vi "AprilTag RoboRIO.vi"() -> ()   [LabVIEW 2023]
uses:
  filter Selector.ctl
  <vilib>/Rock Robotics/WPI/Camera/WPI_CameraImageSize.ctl
  <vilib>/Analysis/baseanly.llb/Real Inverse Matrix.vi
  <vilib>/Analysis/NI_AALBase.lvlib
panel:
  in  "Hilite":bool=TRUE
  in  "Draw Visuals":bool=TRUE
  out "Instructions:":string="Run the VI using the run arrow above. Choose a camera or provided file. Update the tag family to search for. You can change camera resolution on the diagram, outside the loop.\n\nExplore and follow the AprilTag tutorial to explore accuracy and performance tradeoffs. Real-world distance and orientation measurements require tuning the scaling and intrinsic camera matrix beneath the image.\n\nThe white picture to the right is a birds-eye view of a robot with a front-facing camera. The 3D origin is shown at the top-center of the field where the apriltag is attached to that wall.  The charts farther to the right show the YPR and XYZ derived measurements in degrees and inches. Still farther is the detailed info (ID, pixel info, score, and homography matrix)."
  in  "Hamming cutoff":i32
  in  "filter":T1
  out "Y (in)":dbl format="%.1f"
  out "Z (in)":dbl format="%.1f"
  out "X (in)":dbl format="%.1f"
  in  "Length (in)":dbl=100.0
  in  "width (in)":dbl=100.0
  out "Picture":picture
  in  "show rejects":bool
  out "bad":i32
  out "loop time (s)":dbl
  in  "Scale to Inches":dbl[](array[numeric])=[2.5, 2.5, 2.5]
  out "YPR (deg)":cluster{"yaw":dbl, "pitch":dbl, "roll":dbl} {"yaw" format="%.1f"; "pitch" format="%.1f"; "roll" format="%.1f"}
  out "ofsets (in)":cluster{"X":dbl, "Y":dbl, "Z":dbl} {"X" format="%.1f"; "Y" format="%.1f"; "Z" format="%.1f"}
  in  "Intrinsic Camera Matrix":dbl[][](array[numeric])=[[1135.0, 0.0, 640.0], [0.0, 1135.0, 360.0], [0.0, 0.0, 1.0]]
  out "good":i32
  in  "Tag Familys":string[](array[combo])=["16h5"]
  in  "blur":dbl step=0.1
  in  "refine Edges":bool=TRUE
  in  "decimate":dbl=4.0
  in  "threads":i32=1
  out "search time (s)":dbl
  out "good tag details":T2(array[cluster])
  in  "score cutoff":dbl(slide)=60.60606060606061 scale=0.0..100.0
  out "Image":T3(plugin-control)
  # "Offset between\ntarget and camera"
  # "Angles between\ntarget and camera"
  # "Better way to pick camera matrix\ncheck other cams and simplify scaling"
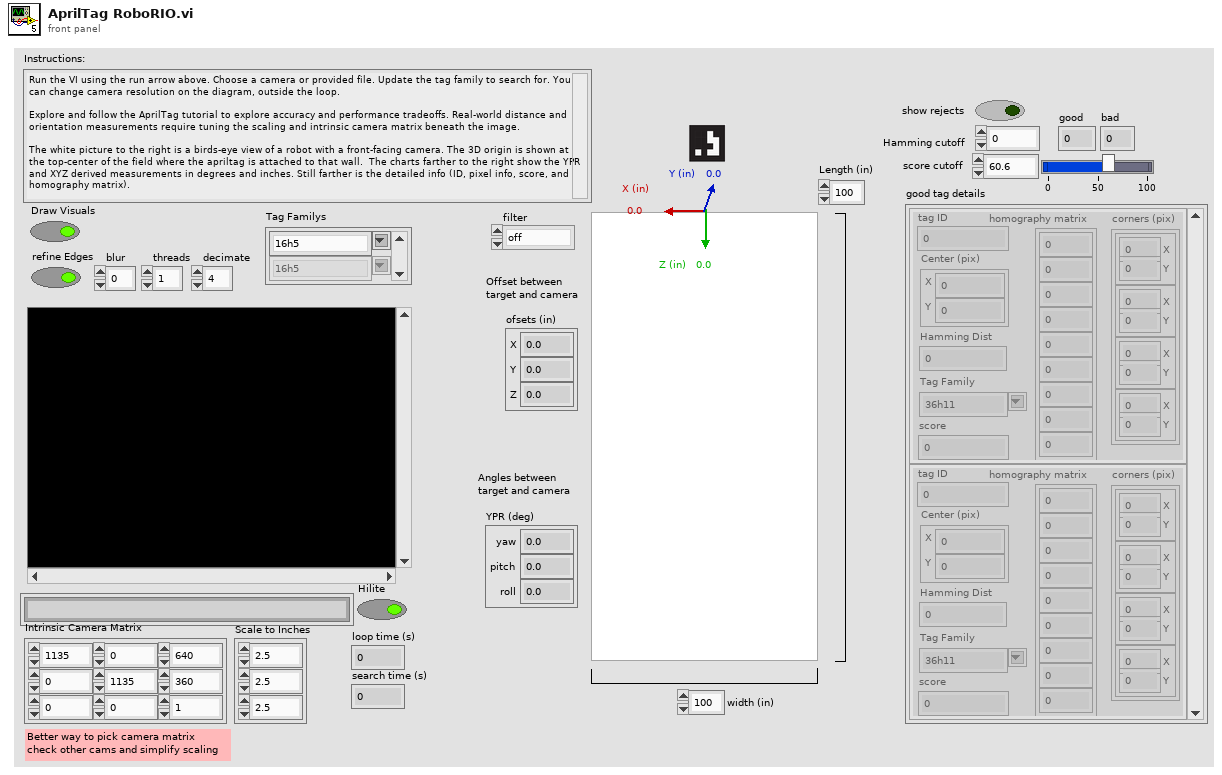
[diagram p1: front panel]
types:
  T1 = typedef "filter Selector.ctl" = enum16{"off", "2 pt avg", "low pass"}
  T2 = cluster{"tag ID":i32, "Center (pix)":cluster{"X":dbl, "Y":dbl}, "homography matrix":dbl[], "score":dbl, "Hamming Dist":i32, "corners (pix)":cluster{"X":dbl, "Y":dbl}[], "Tag Family":string}[]
  T3 = typedef "IMAQ Image.ctl" = refnum<image>
  T4 = typedef "WPI_CameraImageSize.ctl" = enum16{"640x480", "320x240", "160x120", "Custom"}
  T5 = typedef "Image Type" = u32
  T6 = typedef "WPI_CameraDevRef.ctl" = cluster{"Camera Address":string, "CameraStatus":errorcluster}
  T7 = cluster{"tag ID":i32, "Center":cluster{"X":dbl, "Y":dbl}, "homography matrix":dbl[], "decision margin":dbl, "Hamming Dist":i32, "corner points":cluster{"X":dbl, "Y":dbl}[], "Tag Family":string}[]
  T8 = cluster{"Hamming cutoff":i32, "score cutoff":dbl, "show rejects":bool}
  T9 = cluster{"tag ID":i32, "Center":cluster{"X":dbl, "Y":dbl}, "Homography Matrix":dbl[], "dec margin":dbl, "Hamming Dist":i32, "Corner Points":cluster{"X":dbl, "Y":dbl}[], "Tag Family":string}[]
  T10 = typedef "NI_Matrix.lvlib/RealMatrix.ctl" = dbl[][]
  T11 = typedef "LVBoundsTypeDef.ctl" = cluster{"Width":u32, "Height":u32}
  T12 = cluster{"tag ID":i32, "Center":cluster{"X":dbl, "Y":dbl}, "Homography Matrix":dbl[], "dec margin":dbl, "Hamming Dist":i32, "Corner Points":cluster{"X":dbl, "Y":dbl}[], "Tag Family":string}
  T13 = cluster{"Translation[0]":dbl, "Translation[1]":dbl, "Translation[2]":dbl}
  T14 = cluster{"picture out":picture, "offset":cluster{dbl, dbl}}
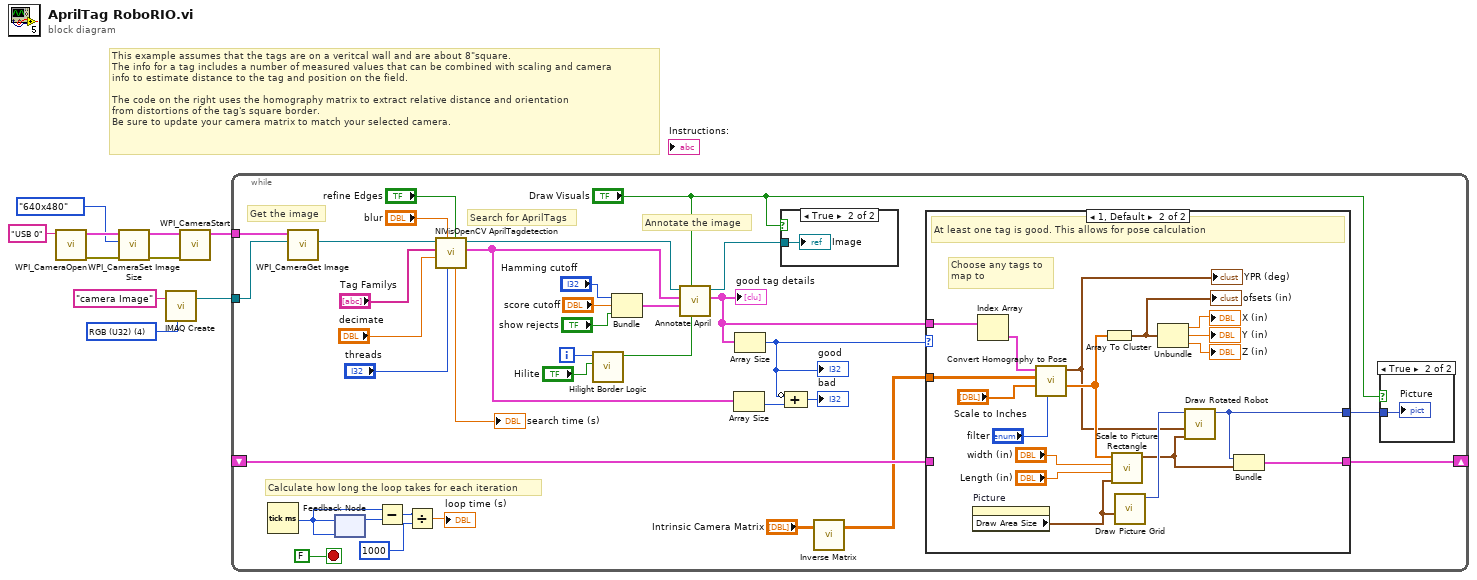
[diagram p0: block diagram]
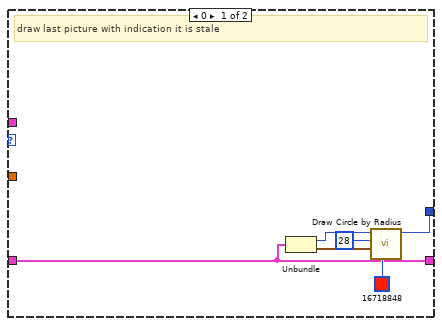
[diagram p4: hidden frame]
diagram:
  w7 = T5 4 items=["Grayscale (U8)", "Grayscale (I16)", "Grayscale (SGL)", "Complex (CSG)", "RGB (U32)", "HSL (U32)", "RGB (U64)", "Grayscale (U16)"] ("Image Type")
  # "This example assumes that the tags are on a veritcal wall and are about 8\"square. \nThe info for a tag includes a number of measured values that can be combined with scaling and camera\ninfo to estimate distance to the tag and position on the field. \n\nThe code on the right uses the homography matrix to extract relative distance and orientation\nfrom distortions of the tag's square border.\nBe sure to update your camera matrix to match your selected camera."
  n1 = call <vilib>:"WPI_CameraOpen.vi"("Camera Address"="USB 0") -> ("error out"=w3:errorcluster, "CameraDevRef"=w5:T6)  [unwired: 9 in]
  n2 = call <vilib>:"WPI_CameraSet Image Size.vi"("error in (no error)"=w3, "Image Size"=WPI_CameraImageSize."640x480", "CameraDevRef"=w5) -> ("error out"=w2:errorcluster, "CameraDevRef Out"=w4:T6)  [unwired: 7 in]
  n3 = call "IMAQ Create"("Image Name"="camera Image", "Image Type"=w7) -> ("New Image"=w6:T3)  [unwired: 3 in, 1 out]
  n4 = call <vilib>:"WPI_CameraStart.vi"("error in (no error)"=w2, "CameraDevRef"=w4) -> ("CameraDevRef"=w9:T6)  [unwired: 8 in, 1 out]
  n5 = while {
    shift-right: [w39] -> _
    shift-left: _ -> [w40]
    tunnel: w9 -> [w15]
    tunnel: w6 -> [w14]
    i -> [w26]
    stop <- FALSE stop-if-true
    # "Calculate how long the loop takes for each iteration"
    # "Annotate the image"
    # "Search for AprilTags"
    # "Get the image"
    n6 = Tick Count (ms)() -> (millisecond timer value=w37:u32)
    n7 = call <vilib>:"WPI_CameraGet Image.vi"("Image"=w14, "CameraDevRef"=w15) -> ("Image Out"=w13:T3)  [unwired: 7 in, 2 out]
    n8 = feedback-in #1(w37) -> ()
    n9 = feedback #1(w37) -> (w38:u32)
    n10 = Subtract(x=w37, y=w38) -> (x-y=w29:u32)
    n11 = Divide(x=w29, y=1000) -> (x/y=→"loop time (s)":dbl)
    n12 = call <vilib>:"NIVisOpenCV AprilTagdetection.vi"("refine Edges"="refine Edges", "threads"="threads", "blur"="blur", "decimate"="decimate", "Tag Familys"="Tag Familys", "Image Src"=w13) -> ("Detected Tags"=w20:T7, "Image Dst Out"=w45:T3, "exec time (s)"=→"search time (s)":dbl)  [unwired: 2 in, 1 out]
    n13 = call "Hilight Border Logic.vi"("Hilight"="Hilite", "index"=w26) -> ("Hilight"=w25:bool)  [unwired: 9 in]
    n14 = Bundle("Hamming cutoff"="Hamming cutoff", "score cutoff"="score cutoff", "show rejects"="show rejects") -> (w21:T8)  [unwired: 1 in]
    n15 = call "Annotate April.vi"("hilight"=w25, "Annotate"="Draw Visuals", "cutoffs"=w21, "Detected Tags"=w20, "Refnum in"=w45) -> ("tags"=w19:T9, "Refnum out"=w44:T3)  [unwired: 4 in, 1 out]
    "good tag details" <- w19
    n16 = Array Size(array=w20) -> (size(s)=w36:i32)
    n17 = Array Size(array=w19) -> (size(s)=w18:i32)
    "good" <- w18
    n18 = case shown="True" "Draw Visuals" {
      tunnel: w44 -> [_ w47]
      frame False {
      }
      frame True {
        "Image" <- w47
      }
    }
    n19 = Compound Arithmetic op=ADD(invert w18, w36) -> (→"bad":i32)
    n20 = call-poly <vilib>:"Inverse Matrix.vi"("Input Matrix"="Intrinsic Camera Matrix") -> ("Inverse Matrix"=w16:T10)  [unwired: 1 in, 1 out]
    n21 = case shown="1, Default" w18 {
      tunnel: w16 -> [_ w71]
      tunnel: [w53 w68] -> w41
      tunnel: w40 -> [w48 _]
      tunnel: [w48 w67] -> w39
      tunnel: w19 -> [_ w66]
      frame 0 {
        # "draw last picture with indication it is stale"
        n22 = Unbundle(w48) -> ("picture out"=w52:picture, "offset"=w51:cluster{dbl, dbl})
        n23 = call <vilib>:"Draw Circle by Radius.vi"("color(black)"=u32 16718848, "pixel center"=w51, "radius"=i16 28, "picture"=w52) -> ("new picture"=w53:picture)  [unwired: 7 in]
      }
      frame 1, Default {
        # "Choose any tags to\nmap to"
        # "At least one tag is good. This allows for pose calculation"
        n24 = property on="Picture" class="Pict"() -> ("Draw Area Size"=w57:T11)  [unwired: 2 in, 2 out]
        n25 = Index Array(array=w66) -> (element=w56:T12)  [unwired: 1 in]
        n26 = call "Convert Homography to Pose.vi"("filter"="filter", "Scale to Inches"="Scale to Inches", "Inverse Camera Matrix"=w71, "tag info"=w56) -> ("Translation"=w58:dbl[], "angles (deg)"=w55:cluster{"yaw":dbl, "pitch":dbl, "roll":dbl})  [unwired: 5 in, 1 out]
        "YPR (deg)" <- w55
        n27 = Array To Cluster(array=w58) -> (cluster=w59:T13)
        "ofsets (in)" <- w59
        n28 = call "Scale to Picture Rectangle.vi"("Draw Area Size"=w57, "Length (in)"="Length (in)", "width (in)"="width (in)", "Translation XYZ"=w58) -> ("offset"=w63:cluster{dbl, dbl})  [unwired: 7 in]
        n29 = call "Draw Picture Grid.vi"("Draw Area Size"=w57) -> ("picture out"=w65:picture)  [unwired: 10 in]
        n30 = Unbundle(w59) -> ("Translation[0]"=→"X (in)":dbl, "Translation[1]"=→"Y (in)":dbl, "Translation[2]"=→"Z (in)":dbl)
        n31 = call "Draw Rotated Robot.vi"("offset"=w63, "YPR (deg)"=w55, "Picture in"=w65) -> ("picture out"=w68:picture)  [unwired: 8 in]
        n32 = Bundle("picture out"=w68, "offset"=w63) -> (w67:T14)  [unwired: 1 in]
      }
    }
    n33 = case shown="True" "Draw Visuals" {
      tunnel: w41 -> [_ w46]
      frame False {
      }
      frame True {
        "Picture" <- w46
      }
    }
  }
